vi "Trap Density_STS.vi"(9 "Temp (T) [K]":dbl, 10 "S.T.S. (S)":dbl, 11 "Dielectric":dbl) -> (3 "Trap Density (N)":dbl)   [LabVIEW 2015]
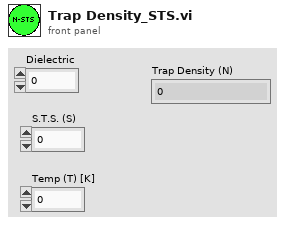
[diagram p1: front panel]
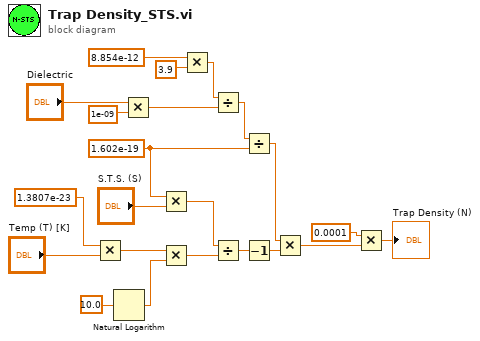
[diagram p0: block diagram]
diagram:
  w22 = 1.602e-19
  n1 = Multiply(x=1.3807e-23, y="Temp (T) [K]") -> (x*y=w17:dbl)
  n2 = Natural Logarithm(1:10.0) -> (0:w16:dbl)
  n3 = Multiply(x="Dielectric", y=1e-09) -> (x*y=w7:dbl)
  n4 = Multiply(x=w22, y="S.T.S. (S)") -> (x*y=w15:dbl)
  n5 = Multiply(x=w17, y=w16) -> (x*y=w14:dbl)
  n6 = Multiply(x=8.854e-12, y=3.9) -> (x*y=w6:dbl)
  n7 = Divide(x=w6, y=w7) -> (x/y=w4:dbl)
  n8 = Divide(x=w15, y=w14) -> (x/y=w13:dbl)
  n9 = Divide(x=w4, y=w22) -> (x/y=w12:dbl)
  n10 = Decrement(x=w13) -> (x-1=w11:dbl)
  n11 = Multiply(x=w12, y=w11) -> (x*y=w3:dbl)
  n12 = Multiply(x=0.0001, y=w3) -> (x*y=→"Trap Density (N)":dbl)
